vi "CRYCreate data header pieces.vi"(11 "x-y settings array":T2=[{"x col"=0, "x data type"=0, "x axis type"=0, "x prefix"="", "x unit"="", "x db ref"=0.0, "y col"=0, "Name:"="", "phase incl"=FALSE, "ym data type"=0, "ym axis type"=0, "ym prefix"="", "ym unit"="", "ym db ref"=0.0, "yp data type"=0, "yp axis type"=0, "yp prefix"="", "yp unit"="", "yp db ref"=0.0}] {"yp db ref" format="%.2f"; "ym db ref" format="%.2f"; "x db ref" format="%.2f"}) -> (3 "Descriptive strings":T1)   [LabVIEW 2013]
uses:
  Control/CRYx-y settings array.ctl
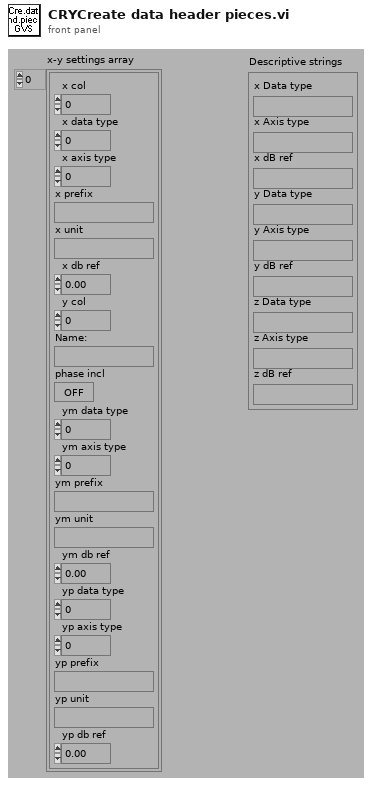
[diagram p1: front panel]
types:
  T1 = cluster{"x Data type":string, "x Axis type":string, "x dB ref":string, "y Data type":string, "y Axis type":string, "y dB ref":string, "z Data type":string, "z Axis type":string, "z dB ref":string}
  T2 = typedef "CRYx-y settings array.ctl" = cluster{"x col":i32, "x data type":u16, "x axis type":u16, "x prefix":string, "x unit":string, "x db ref":dbl, "y col":i32, "Name:":string, "phase incl":bool, "ym data type":u16, "ym axis type":u16, "ym prefix":string, "ym unit":string, "ym db ref":dbl, "yp data type":u16, "yp axis type":u16, "yp prefix":string, "yp unit":string, "yp db ref":dbl}[]
  T3 = cluster{"x col":i32, "x data type":u16, "x axis type":u16, "x prefix":string, "x unit":string, "x db ref":dbl, "y col":i32, "Name:":string, "phase incl":bool, "ym data type":u16, "ym axis type":u16, "ym prefix":string, "ym unit":string, "ym db ref":dbl, "yp data type":u16, "yp axis type":u16, "yp prefix":string, "yp unit":string, "yp db ref":dbl}
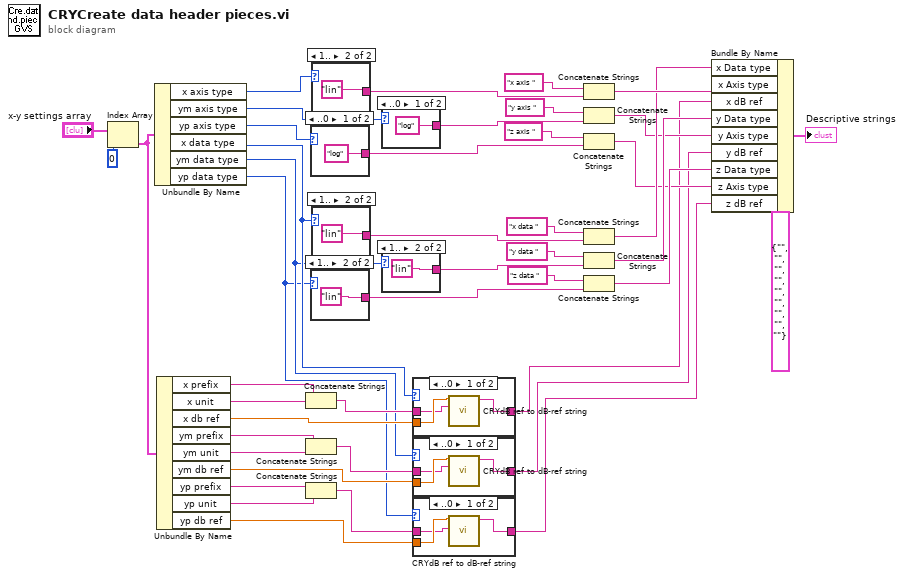
[diagram p0: block diagram]
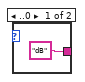
[diagram p2: hidden frame]
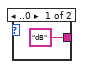
[diagram p3: hidden frame]
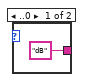
[diagram p4: hidden frame]
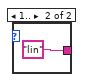
[diagram p8: hidden frame]
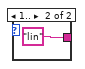
[diagram p9: hidden frame]
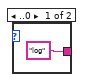
[diagram p10: hidden frame]
diagram:
  n1 = Index Array(array="x-y settings array", index=0 ("Index")) -> (element=w41:T3)
  n2 = Unbundle By Name(w41) -> ("x axis type"=w44:u16, "ym axis type"=w43:u16, "yp axis type"=w42:u16, "x data type"=w28:u16, "ym data type"=w27:u16, "yp data type"=w26:u16)
  n3 = Unbundle By Name(w41) -> ("x prefix"=w40:string, "x unit"=w39:string, "x db ref"=w33:dbl, "ym prefix"=w38:string, "ym unit"=w37:string, "ym db ref"=w31:dbl, "yp prefix"=w36:string, "yp unit"=w35:string, "yp db ref"=w29:dbl)
  n4 = Concatenate Strings(w40, w39) -> (w34:string)
  n5 = Concatenate Strings(w38, w37) -> (w32:string)
  n6 = Concatenate Strings(w36, w35) -> (w30:string)
  n7 = case shown="..0" w42 {
    tunnel: ["log" "lin"] -> w16
    frame ..0 {
    }
    frame 1.. {
    }
  }
  n8 = case shown="1.." w26 {
    tunnel: ["dB" "lin"] -> w10
    frame ..0 {
    }
    frame 1.. {
    }
  }
  n9 = case shown="1.." w44 {
    tunnel: ["log" "lin"] -> w20
    frame ..0 {
    }
    frame 1.. {
    }
  }
  n10 = case shown="1.." w28 {
    tunnel: ["dB" "lin"] -> w14
    frame ..0 {
    }
    frame 1.. {
    }
  }
  n11 = case shown="..0" w43 {
    tunnel: ["log" "lin"] -> w18
    frame ..0 {
    }
    frame 1.. {
    }
  }
  n12 = case shown="1.." w27 {
    tunnel: ["dB" "lin"] -> w12
    frame ..0 {
    }
    frame 1.. {
    }
  }
  n13 = case shown="..0" w28 {
    tunnel: w34 -> [w57 w60]
    tunnel: w33 -> [w59 _]
    tunnel: [w58 w60] -> w3
    frame ..0 {
      n14 = call "CRYdB ref to dB-ref string.vi"("base prefix/unit"=w57, "dB ref"=w59) -> ("dB/ref string"=w58:string)  [unwired: 5 in]
    }
    frame 1.. {
    }
  }
  n15 = case shown="..0" w27 {
    tunnel: w32 -> [w61 w64]
    tunnel: w31 -> [w63 _]
    tunnel: [w62 w64] -> w2
    frame ..0 {
      n16 = call "CRYdB ref to dB-ref string.vi"("base prefix/unit"=w61, "dB ref"=w63) -> ("dB/ref string"=w62:string)  [unwired: 5 in]
    }
    frame 1.. {
    }
  }
  n17 = case shown="..0" w26 {
    tunnel: w30 -> [w65 w68]
    tunnel: w29 -> [w67 _]
    tunnel: [w66 w68] -> w1
    frame ..0 {
      n18 = call "CRYdB ref to dB-ref string.vi"("base prefix/unit"=w65, "dB ref"=w67) -> ("dB/ref string"=w66:string)  [unwired: 5 in]
    }
    frame 1.. {
    }
  }
  n19 = Concatenate Strings("x axis ", w20) -> (w9:string)
  n20 = Concatenate Strings("y axis ", w18) -> (w5:string)
  n21 = Concatenate Strings("z axis ", w16) -> (w4:string)
  n22 = Concatenate Strings("x data ", w14) -> (w8:string)
  n23 = Concatenate Strings("y data ", w12) -> (w7:string)
  n24 = Concatenate Strings("z data ", w10) -> (w6:string)
  n25 = Bundle By Name(cluster=T1 {"x Data type"="", "x Axis type"="", "x dB ref"="", "y Data type"="", "y Axis type"="", "y dB ref"="", "z Data type"="", "z Axis type"="", "z dB ref"=""} ("Descriptive strings"), "x Data type"=w8, "x Axis type"=w9, "x dB ref"=w3, "y Data type"=w7, "y Axis type"=w5, "y dB ref"=w2, "z Data type"=w6, "z Axis type"=w4, "z dB ref"=w1) -> (→"Descriptive strings":T1)
